vi "더하기.vi"() -> ()   [LabVIEW 2014]
panel:
  out "숫자형 3":dbl
  in  "숫자형 2":dbl
  in  "숫자형":dbl
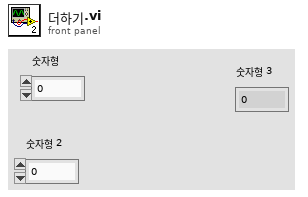
[diagram p1: front panel]
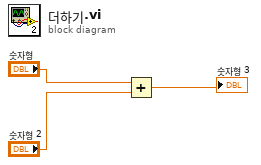
[diagram p0: block diagram]
diagram:
  n1 = Add(x="숫자형", y="숫자형 2") -> (x+y=→"숫자형 3":dbl)
